vi "Read Delay.vi"(8 "error in (no error)":errorcluster, 11 "Action Step in":refnum<class "Action Step.lvclass">) -> (0 "error out":errorcluster, 2 "Delay":i32, 3 "Action Step out":refnum<class "Action Step.lvclass">)   [LabVIEW 2020, in "MacroAssert.lvlib" / "Action Step.lvclass"]
uses:
  Action Step.lvclass
  Action Step.lvclass/Action Step.ctl
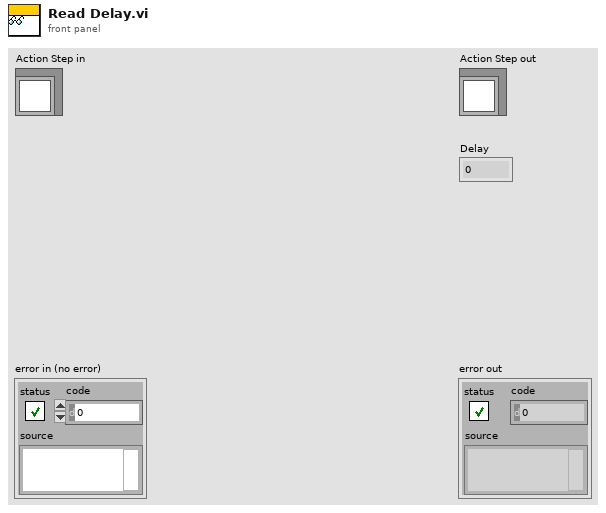
[diagram p1: front panel]
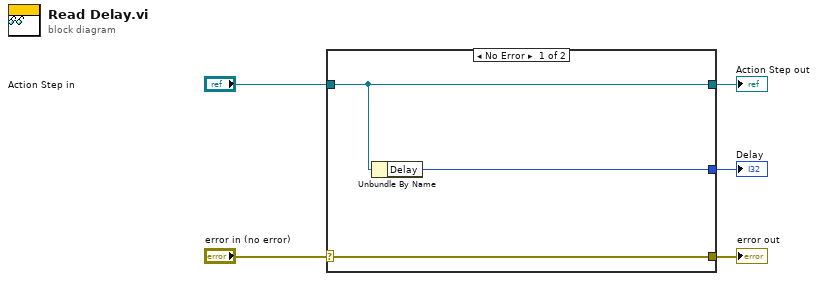
[diagram p0: block diagram]
diagram:
  n1 = case shown="No Error" "error in (no error)" {
    selector: "error in (no error)" -> [w8 w9]
    tunnel: [w8 w9] -> w4
    tunnel: [w7 w10] -> w2
    tunnel: "Action Step in" -> [w7 w10]
    tunnel: [w6 _] -> w1
    frame No Error {
      n2 = Unbundle By Name(w7) -> ("Delay"=w6:i32)
    }
    frame Error {
    }
  }
  "error out" <- w4
  "Action Step out" <- w2
  "Delay" <- w1
